vi "close configuration file.vi"(8 "error in (no error)":errorcluster, 11 "Configuration File in":refnum<class "Configuration File.lvclass">) -> (0 "error out":errorcluster, 3 "Configuration File out":refnum<class "Configuration File.lvclass">)   [LabVIEW 2018, in "Configuration File.lvclass"]
uses:
  Configuration File.lvclass
  Configuration File.lvclass/Configuration File.ctl
  <vilib>/Utility/config.llb/NI_LVConfig.lvlib
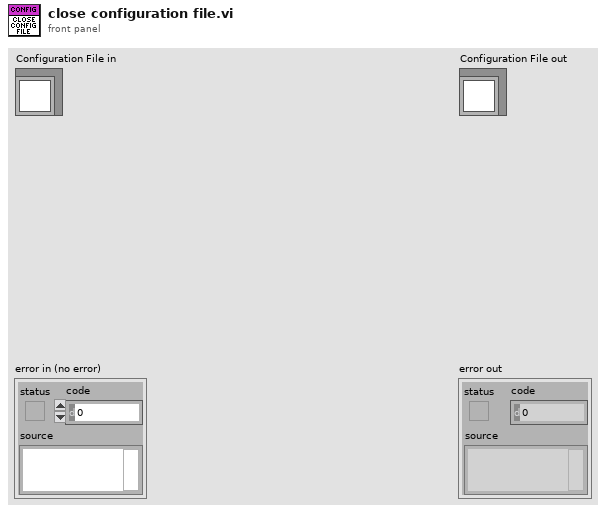
[diagram p1: front panel]
types:
  T1 = typedef "NI_LVConfig.lvlib/Config Data RefNum.ctl" = refnum<k1>
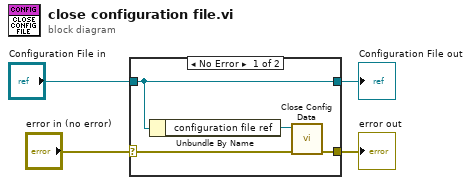
[diagram p0: block diagram]
diagram:
  n1 = case shown="No Error" "error in (no error)" {
    selector: "error in (no error)" -> [w8 w10]
    tunnel: [w7 w10] -> w3
    tunnel: [w6 w9] -> w1
    tunnel: "Configuration File in" -> [w6 w9]
    frame No Error {
      n2 = Unbundle By Name(w6) -> ("configuration file ref"=w5:T1)
      n3 = call <vilib>:"Close Config Data.vi"("error in (no error)"=w8, "refnum"=w5) -> ("error out"=w7:errorcluster)  [unwired: 8 in, 1 out]
    }
    frame Error {
    }
  }
  "error out" <- w3
  "Configuration File out" <- w1
